vi "Analysis.GetCycledChannels.vi"(8 "error in (no error)":errorcluster, 11 "Data":path) -> (0 "error out":errorcluster, 1 "DUTs":string[](array[string]), 2 "Cycled":bool[](array[boolean]))   [LabVIEW 2014, in "NIAnalysis.lvlib"]
uses:
  NIAnalysis.lvlib
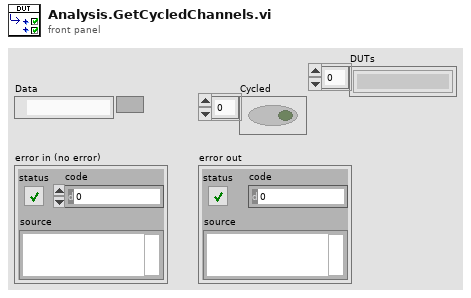
[diagram p1: front panel]
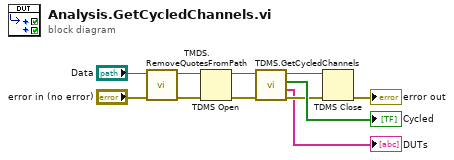
[diagram p0: block diagram]
diagram:
  n1 = call "TMDS.RemoveQuotesFromPath.vi"("error in (no error)"="error in (no error)", "Data"="Data") -> ("error out"=w5:errorcluster, "Path"=w3:path)  [unwired: 8 in]
  n2 = TDMS Open(8:w5, 11:w3) -> (0:w6:errorcluster, 3:w7:refnum<k34>)  [unwired: 5 in]
  n3 = call "TDMS.GetCycledChannels.vi"("error in (no error)"=w6, "TDMS Ref"=w7) -> ("error out"=w8:errorcluster, "DUTs"=→"DUTs":string[], "Cycled"=→"Cycled":bool[], "TDMS Ref"=w9:refnum<k34>)  [unwired: 6 in]
  n4 = TDMS Close(8:w8, 11:w9) -> (0:→"error out":errorcluster)  [unwired: 1 out]
